vi "counter_event_v2.vi"() -> ()   [LabVIEW 2019]
panel:
  in  "Reset":bool
  in  "stop":bool
  out "Count":u32
  in  "Button":bool
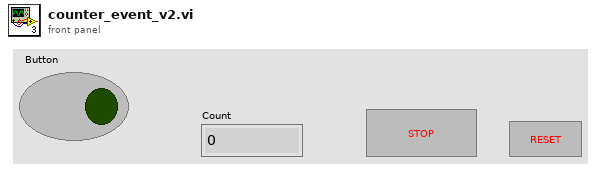
[diagram p1: front panel]
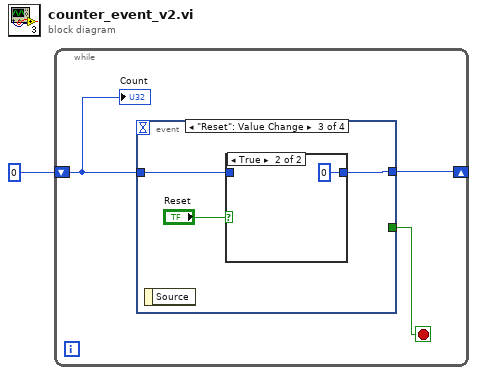
[diagram p0: block diagram]
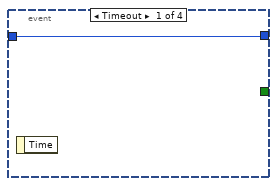
[diagram p2: hidden frame]
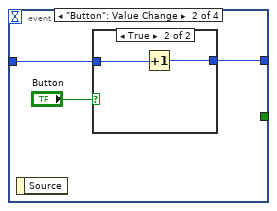
[diagram p3: hidden frame]
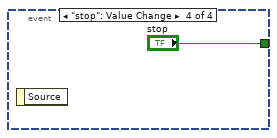
[diagram p6: hidden frame]
diagram:
  n1 = while {
    shift-right: [w3] -> _
    shift-left: u32 0 ("milliseconds to wait") -> [w4]
    stop <- w2 stop-if-true
    n2 = event shown="[2] \"Reset\": Value Change" {
      selector: _ -> [_ _ _ _]
      dyn-events: _ -> [_ _ _ _]
      timeout: _ -> [_ _ _ _]
      tunnel: w4 -> [w5 w7 w13 _]
      tunnel: [w5 w6 w12 _] -> w3
      tunnel: [_ _ _ "stop"] -> w2
      event Timeout {
        n3 = event-data() -> ()  [unwired: 1 in, 1 out]
      }
      event "Button": Value Change {
        n4 = event-data() -> ()  [unwired: 1 in, 1 out]
        n5 = case shown="True" "Button" {
          tunnel: w7 -> [w9 w11]
          tunnel: [w9 w10] -> w6
          frame False {
          }
          frame True {
            n6 = Increment(x=w11) -> (x+1=w10:u32)
          }
        }
      }
      event "Reset": Value Change {
        n7 = event-data() -> ()  [unwired: 1 in, 1 out]
        n8 = case shown="True" "Reset" {
          tunnel: w13 -> [w15 _]
          tunnel: [w15 u32 0 ("milliseconds to wait")] -> w12
          frame False {
          }
          frame True {
          }
        }
      }
      event "stop": Value Change {
        n9 = event-data() -> ()  [unwired: 1 in, 1 out]
      }
    }
    "Count" <- w4
  }
